vi "LabVIEW Blowfish Encryption.vi"(0 "Password":string, 1 "Enc/Dec":enum16{"Encipher", "Decipher"}(ring), 2 "Input Text":string, 4 "Output As ASCII\nfor email Transmission":bool, 5 "error in (no error)":errorcluster) -> (6 "Output text":string, 7 "Compression Ratio":dbl=1.0, 8 "error out":errorcluster)   [LabVIEW 2020, in "Registration.lvclass"]
doc: "The Blowfish Encryption Algorithm\n\nBlock cipher: 64-bit block \nVariable key length: 32 bits to 448 bits \nDesigned by Bruce Schneier \nMuch faster than DES and IDEA \nUnpatented and royalty-free \nNo license required \n\nBlowfish is a symmetric block cipher that can be used as a drop-in replacement for DES or IDEA. It takes a variable-length key, from 32 bits to 448 bits, making it ideal for both domestic and exportable use. Blowfish was designed in 1993 by Bruce Schneier as a fast, free alternative to existing encryption algorithms. Since then it has been analyzed considerably, and it is slowly gaining acceptance as a strong encryption algorithm. Blowfish is unpatented and license-free, and is available free for all uses.\n\nAs far as I know this is the first implementation of the Blowfish Algorithm in LabVIEW. With this set of subvi's one can encrypt data in LabVIEW without the need of external software. This can be used to send data securely over Data socket as well as TCP and UDP communications. And also protect remote control systems from unauthorized access, by encrypting the control communications.\n\nI welcome any constructive commits, and bug reports can be sent to the E-mail contained in the code"
uses:
  Registration.lvclass
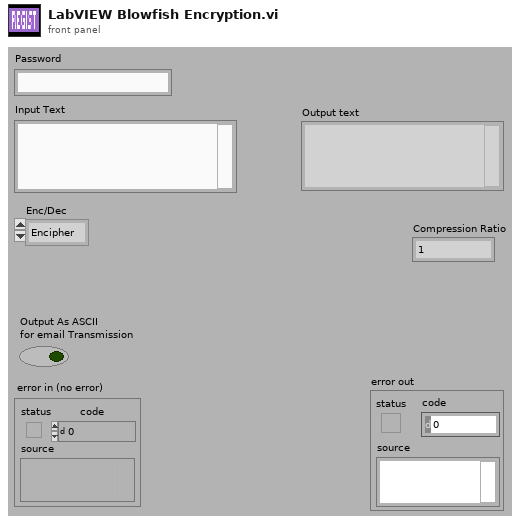
[diagram p1: front panel]
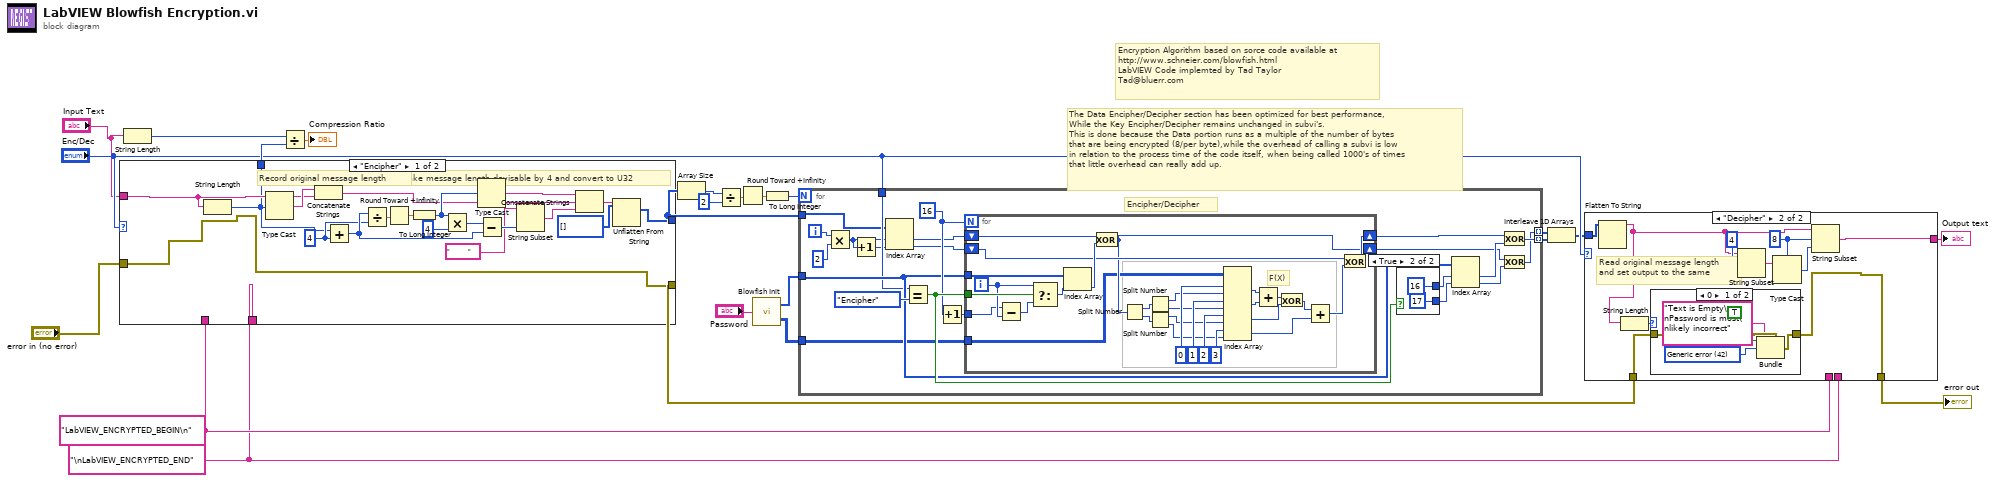
[diagram p0: block diagram]
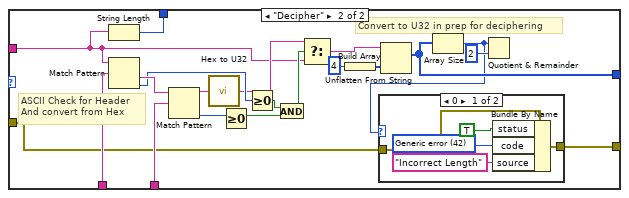
[diagram p2: hidden frame]
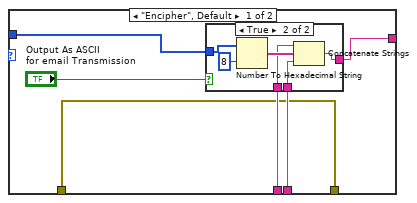
[diagram p4: hidden frame]
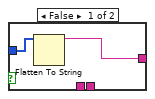
[diagram p5: hidden frame]
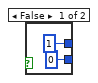
[diagram p7: hidden frame]
diagram:
  w6 = "\nLabVIEW_ENCRYPTED_END"
  w7 = "LabVIEW_ENCRYPTED_BEGIN\n"
  # "Encryption Algorithm based on sorce code available at\nhttp://www.schneier.com/blowfish.html\nLabVIEW Code implemted by Tad Taylor\nTad@bluerr.com"
  # "The Data Encipher/Decipher section has been optimized for best performance,\nWhile the Key Encipher/Decipher remains unchanged in subvi's.\nThis is done because the Data portion runs as a multiple of the number of bytes\nthat are being encrypted (8/per byte),while the overhead of calling a subvi is low\nin relation to the process time of the code itself, when being called 1000's of times\nthat little overhead can really add up."
  n1 = case shown="\"Encipher\"" "Enc/Dec" {
    tunnel: "Input Text" -> [w27 w47]
    tunnel: [w28 w59] -> w1
    tunnel: [w26 w58] -> w12
    tunnel: w7 -> [_ w55]
    tunnel: w6 -> [_ w54]
    tunnel: "error in (no error)" -> [w25 w45]
    tunnel: [w25 w44] -> w3
    frame "Encipher" {
      w32 = 4 ("y")
      # "Make message length devisable by 4 and convert to U32"
      # "Record original message length"
      n2 = String Length(string=w27) -> (length=w26:i32)
      n3 = Type Cast(x=w26) -> (*(type *) &x=w29:string)  [unwired: 1 in]
      n4 = Concatenate Strings(w29, w27) -> (w35:string)
      n5 = Add(x=w26, y=w32) -> (x+y=w42:i32)
      n6 = Divide(x=w42, y=w32) -> (x/y=w30:dbl)
      n7 = Round Toward +Infinity(x=w30) -> (ceil(x): smallest int >= x=w31:dbl)
      n8 = To Long Integer(number=w31) -> (32bit integer=w36:i32)
      n9 = Multiply(x=w36, y=4) -> (x*y=w38:i32)
      n10 = Type Cast(x=w36) -> (*(type *) &x=w33:string)  [unwired: 1 in]
      n11 = Subtract(x=w38, y=w42) -> (x-y=w40:i32)
      n12 = String Subset(string="         ", length (rest)=w40) -> (substring=w41:string)  [unwired: 1 in]
      n13 = Concatenate Strings(w33, w35, w41) -> (w34:string)
      n14 = Unflatten From String(type=u32[] [] ("appended array"), binary string=w34) -> (value=w28:u32[])  [unwired: 3 in, 2 out]
    }
    frame "Decipher" {
      # "Convert to U32 in prep for deciphering"
      # "ASCII Check for Header\nAnd convert from Hex"
      n15 = String Length(string=w47) -> (length=w58:i32)
      n16 = Match Pattern(string=w47, regular expression=w55) -> (after substring=w56:string, offset past match=w52:i32)  [unwired: 1 in, 2 out]
      n17 = Match Pattern(string=w56, regular expression=w54) -> (before substring=w57:string, offset past match=w53:i32)  [unwired: 1 in, 2 out]
      n18 = call "Hex to U32.vi"("Hex"=w57) -> ("U32"=w48:string)
      n19 = Greater Or Equal To 0?(x=w53) -> (x >= 0?=w50:bool)
      n20 = Greater Or Equal To 0?(x=w52) -> (x >= 0?=w51:bool)
      n21 = And(x=w51, y=w50) -> (x .and. y?=w49:bool)
      n22 = Select(t=w48, s=w49, f=w47) -> (s? t:f=w46:string)
      n23 = Build Array(u32 4 ("offset (0)")) -> (w61:u32[])
      n24 = Unflatten From String(type=w61, binary string=w46) -> (value=w59:u32[])  [unwired: 3 in, 2 out]
      n25 = Array Size(array=w59) -> (size(s)=w43:i32)
      n26 = case shown="0" w43 {
        tunnel: w45 -> [w67 w68]
        tunnel: [w66 w68] -> w44
        frame 0 {
          w63 = 42 items=["No error", "Argument error", "Memory is full", "Out of zone", "End of file", "File already open", "Generic file I/O error", "File not found", "File permission error", "Disk is full", "Duplicate path", "Too many files open", "System feature not enabled", "Resource file not found", "Cannot add resource", "Resource not found", "Image not found", "Image memory error", "Pen does not exist", "Config type invalid", "Config token not found", "Config parse error", "Config memory error", "Bad external code format", "Bad external code offset", "External code not present", "Null window", "Destroy window error", "Null menu", "Print aborted", "Bad print record", "Print driver error", "Windows error during printing", "Memory error during printing", "Print dialog error", "Generic print error", "Invalid device refnum", "Device not found", "Device parameter error", "Device unit error", "Cannot open device", "Device call aborted", "Generic error", "Cancelled by user", "Object ID too low", "Object ID too high", "Object not in heap", "Unknown heap", "Unknown object (invalid DefProc)", "Unknown object (DefProc not in table)", "Message out of range", "Invalid (null) method", "Unknown message", "Manager call not supported", "Bad address", "Network operation in progress", "Network operation timed out", "Connection is busy", "Network attribute not supported", "Network error", "Address in use", "System out of memory", "Connection aborted", "Connection refused", "Not connected", "Already connected", "Connection closed", "Initialization error (interapplication manager)", "Bad occurrence", "Wait on unbound occurrence handler", "Occurrence queue overflow", "Datalog type conflict", "Unused", "Unrecognized type (interapplication manager)", "Memory corrupt", "Failed to make temporary DLL", "Old CIN version", "Drag socket not found", "Failed to load drop-object", "Failed to register OLE object", "Failed to release OLE object", "Format specifier type mismatch", "Unknown format specifier", "Too few format specifiers", "Too many format specifiers", "Scan failed", "Newer CIN version", "Error converting to variant", "Runtime menu error", "Password tampered", "Variant attribute not found", "Incompatible variant data type", "Event data is not available", "Event Store is not present", "Occurrence is not found", "Event Queue is not created", "Event info is not available", "Refnum passed is NULL", "Error retrieving Class GUID", "Error retrieving CoClass GUID", "Error retrieving TypeLib GUID.", "Bad built application magic bytes.", "Specific driver is different from the specific driver associated with the Logical Name.", "There is no session opened to the class driver.", "Max Error", "MAX - Error with config objects", "MAX - Error loading configuration", "MAX - Group not supported"]
          n27 = Bundle By Name(cluster=w67, "status"=TRUE, "code"=w63, "source"="Incorrect Length") -> (w66:errorcluster)
        }
        frame 1, Default {
        }
      }
      n28 = Quotient & Remainder(x=w43, y=2) -> ()  [unwired: 2 out]
    }
  }
  n29 = String Length(string="Input Text") -> (length=w13:i32)
  n30 = Divide(x=w13, y=w12) -> (x/y=→"Compression Ratio":dbl)
  n31 = Array Size(array=w1) -> (size(s)=w15:i32)
  n32 = Divide(x=w15, y=2 ("x")) -> (x/y=w17:dbl)
  n33 = Round Toward +Infinity(x=w17) -> (ceil(x): smallest int >= x=w18:dbl)
  n34 = call "Blowfish Init.vi"("Key"="Password") -> ("P 18"=w22:u32[], "S 4X256"=w21:u32[][])
  n35 = To Long Integer(number=w18) -> (32bit integer=w14:i32)
  n36 = for {
    N: w14 -> [_]
    tunnel: "Enc/Dec" -> [w78]
    tunnel: [w79] -> w20 mode=indexing
    tunnel: [w80] -> w19 mode=indexing
    tunnel: w22 -> [w82]
    tunnel: w21 -> [w81]
    tunnel: w1 -> [w75]
    i -> [w74]
    w87 = 16
    # "Encipher/Decipher"
    n37 = Multiply(x=w74, y=u32 2 ("element")) -> (x*y=w72:u32)
    n38 = Increment(x=w72) -> (x+1=w73:u32)
    n39 = Index Array(array=w75, index #1=w72, index #2=w73) -> (element #1=w70:u32, element #2=w71:u32)
    n40 = Equal?(x=w78, y=enum16{"Encipher", "Decipher"}."Encipher") -> (x = y?=w90:bool)
    n41 = Increment(x=w87) -> (x+1=w86:i32)
    n42 = for {
      N: w87 -> [_]
      shift-right: [w114] -> w77
      shift-left: w70 -> [w116]
      tunnel: w82 -> [w123]
      tunnel: w81 -> [w96]
      tunnel: w90 -> [w121]
      tunnel: w86 -> [w117]
      shift-right: [w97] -> w76
      shift-left: w71 -> [w115]
      i -> [w118]
      # "F(X)"
      n43 = Subtract(x=w117, y=w118) -> (x-y=w119:i32)
      n44 = Select(t=w118, s=w121, f=w119) -> (s? t:f=w120:i32)
      n45 = Index Array(array=w123, index=w120) -> (element=w122:u32)
      n46 = Exclusive Or(1:w122, 2:w116) -> (0:w97:u32)
      n47 = Split Number(x=w97) -> (hi(x)=w113:u16, lo(x)=w112:u16)
      n48 = Split Number(x=w113) -> (hi(x)=w101:u8, lo(x)=w100:u8)
      n49 = Split Number(x=w112) -> (hi(x)=w99:u8, lo(x)=w98:u8)
      n50 = Index Array(array=w96, index (row) #1=0 ("index (row)"), index (col) #1=w101, index (row) #2=1 ("index (row)"), index (col) #2=w100, index (row) #3=2 ("index (row)"), index (col) #3=w99, index (row) #4=3 ("index (row)"), index (col) #4=w98) -> (element #1=w107:u32, element #2=w106:u32, element #3=w104:u32, element #4=w102:u32)
      n51 = Add(x=w107, y=w106) -> (x+y=w105:u32)
      n52 = Exclusive Or(1:w104, 2:w105) -> (0:w103:u32)
      n53 = Add(x=w103, y=w102) -> (x+y=w95:u32)
      n54 = Exclusive Or(1:w95, 2:w115) -> (0:w114:u32)
    }
    n55 = case shown="True" w90 {
      tunnel: [0 ("f") 17 ("f")] -> w88
      tunnel: [1 ("f") 16 ("f")] -> w89
      frame False {
      }
      frame True {
      }
    }
    n56 = Index Array(array=w82, index #1=w89, index #2=w88) -> (element #1=w84:u32, element #2=w83:u32)
    n57 = Exclusive Or(1:w84, 2:w77) -> (0:w80:u32)
    n58 = Exclusive Or(1:w83, 2:w76) -> (0:w79:u32)
  }
  n59 = Interleave 1D Arrays(w20, w19) -> (w8:u32[])
  n60 = case shown="\"Decipher\"" "Enc/Dec" {
    tunnel: [w127 w138] -> w9
    tunnel: w8 -> [w128 w143]
    tunnel: w7 -> [w126 _]
    tunnel: w6 -> [w125 _]
    tunnel: w3 -> [w124 w140]
    tunnel: [w124 w139] -> w2
    frame "Encipher", Default {
      n61 = case shown="True" "Output As ASCII\nfor email Transmission" {
        tunnel: [w131 w135] -> w127
        tunnel: w128 -> [w130 w134]
        tunnel: w126 -> [_ w133]
        tunnel: w125 -> [_ w132]
        frame False {
          n62 = Flatten To String(anything=w130) -> (data string=w131:string)  [unwired: 3 in, 2 out]
        }
        frame True {
          n63 = Number To Hexadecimal String(1:i16 8 ("width (-)"), 2:w134) -> (0:w136:string[])
          n64 = Concatenate Strings(w133, w136, w132) -> (w135:string)
        }
      }
    }
    frame "Decipher" {
      w147 = 4 ("offset (0)")
      w145 = 8 ("offset (0)")
      # "Read original message length\nand set output to the same"
      n65 = Flatten To String(anything=w143) -> (data string=w141:string)  [unwired: 3 in, 2 out]
      n66 = String Length(string=w141) -> (length=w142:i32)
      n67 = case shown="0" w142 {
        tunnel: w140 -> [w152 w153]
        tunnel: [w149 w153] -> w139
        frame 0 {
          w148 = 42 items=["No error", "Argument error", "Memory is full", "Out of zone", "End of file", "File already open", "Generic file I/O error", "File not found", "File permission error", "Disk is full", "Duplicate path", "Too many files open", "System feature not enabled", "Resource file not found", "Cannot add resource", "Resource not found", "Image not found", "Image memory error", "Pen does not exist", "Config type invalid", "Config token not found", "Config parse error", "Config memory error", "Bad external code format", "Bad external code offset", "External code not present", "Null window", "Destroy window error", "Null menu", "Print aborted", "Bad print record", "Print driver error", "Windows error during printing", "Memory error during printing", "Print dialog error", "Generic print error", "Invalid device refnum", "Device not found", "Device parameter error", "Device unit error", "Cannot open device", "Device call aborted", "Generic error", "Cancelled by user", "Object ID too low", "Object ID too high", "Object not in heap", "Unknown heap", "Unknown object (invalid DefProc)", "Unknown object (DefProc not in table)", "Message out of range", "Invalid (null) method", "Unknown message", "Manager call not supported", "Bad address", "Network operation in progress", "Network operation timed out", "Connection is busy", "Network attribute not supported", "Network error", "Address in use", "System out of memory", "Connection aborted", "Connection refused", "Not connected", "Already connected", "Connection closed", "Initialization error (interapplication manager)", "Bad occurrence", "Wait on unbound occurrence handler", "Occurrence queue overflow", "Datalog type conflict", "Unused", "Unrecognized type (interapplication manager)", "Memory corrupt", "Failed to make temporary DLL", "Old CIN version", "Drag socket not found", "Failed to load drop-object", "Failed to register OLE object", "Failed to release OLE object", "Format specifier type mismatch", "Unknown format specifier", "Too few format specifiers", "Too many format specifiers", "Scan failed", "Newer CIN version", "Error converting to variant", "Runtime menu error", "Password tampered", "Variant attribute not found", "Incompatible variant data type", "Event data is not available", "Event Store is not present", "Occurrence is not found", "Event Queue is not created", "Event info is not available", "Refnum passed is NULL", "Error retrieving Class GUID", "Error retrieving CoClass GUID", "Error retrieving TypeLib GUID.", "Bad built application magic bytes.", "Specific driver is different from the specific driver associated with the Logical Name.", "There is no session opened to the class driver.", "Max Error", "MAX - Error with config objects", "MAX - Error loading configuration", "MAX - Group not supported"]
          n68 = Bundle(cluster=w152, "status"=TRUE, "code"=w148, "source"="Text is Empty\nPassword is most\nlikely incorrect") -> (w149:errorcluster)
        }
        frame 1, Default {
        }
      }
      n69 = String Subset(string=w141, offset (0)=w147, length (rest)=w147) -> (substring=w146:string)
      n70 = Type Cast(type=w145, x=w146) -> (*(type *) &x=w144:i32)
      n71 = String Subset(string=w141, offset (0)=w145, length (rest)=w144) -> (substring=w138:string)
    }
  }
  "Output text" <- w9
  "error out" <- w2
